vi "Güç_Tablo_Doldur.vi"(10 "Table Reference in":refnum<vi>, 11 "Array In":dbl[][](array[numeric])) -> (1 "Test Result":bool, 2 "Table Values":string[][](array[string]), 3 "Array Out":dbl[][](array[numeric]))   [LabVIEW 2014]
uses:
  TestStandInteraction/VeriPaylasim_Globali.vi
panel:
  out "OlcumNo":u16
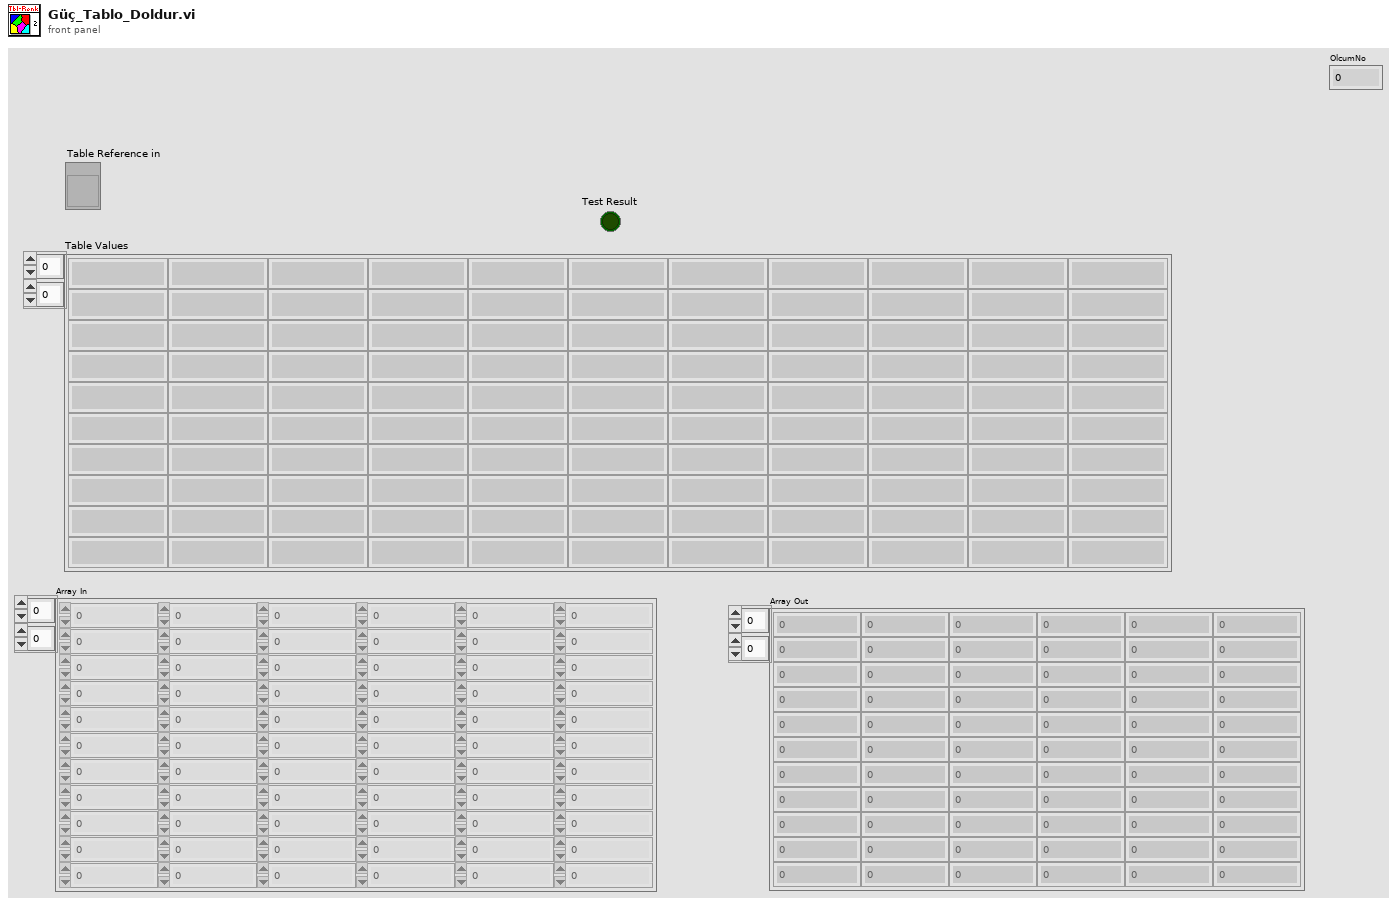
[diagram p1: front panel]
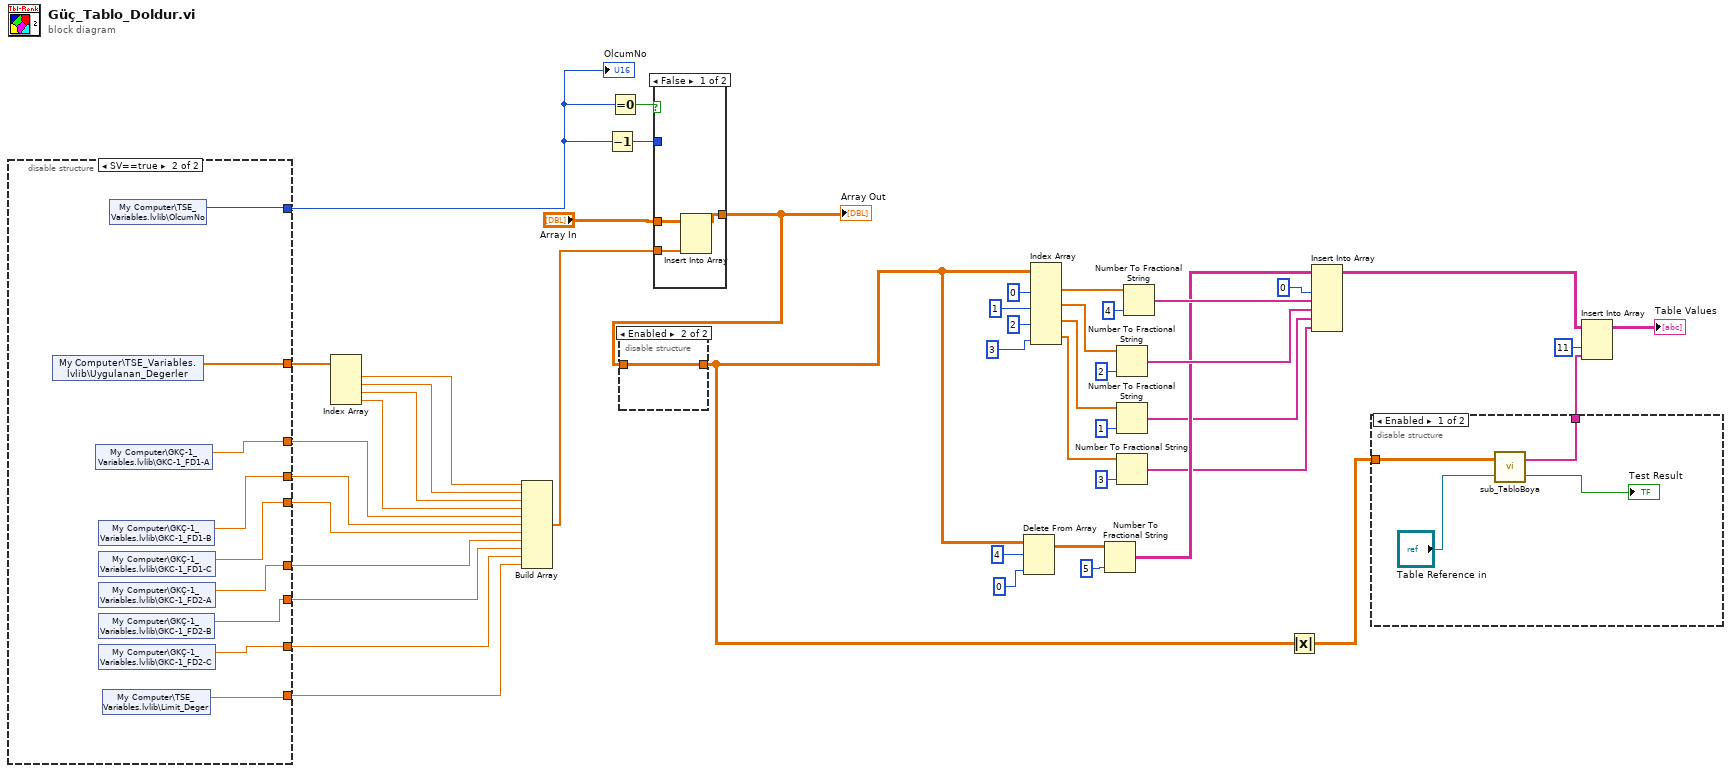
[diagram p0: block diagram]
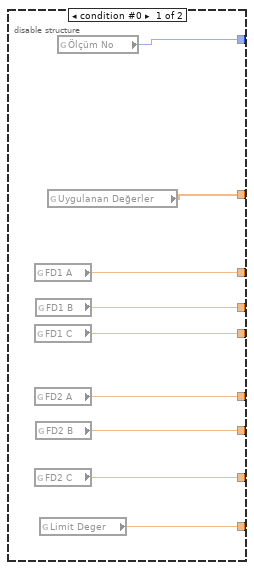
[diagram p2: hidden frame]
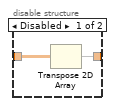
[diagram p3: hidden frame]
diagram:
  n1 = disable-structure shown="SV==true" {
    disable-tunnel: [w55 w57] -> w43
    disable-tunnel: [w54 w58] -> w8
    disable-tunnel: [w53 w59] -> w7
    disable-tunnel: [w52 w60] -> w6
    disable-tunnel: [w51 w61] -> w5
    disable-tunnel: [w50 w62] -> w4
    disable-tunnel: [w49 w63] -> w3
    disable-tunnel: [w48 w64] -> w2
    disable-tunnel: [w47 w56] -> w1
    frame condition #0 {
      n2 = global read "VeriPaylasim_Globali.vi" "FD1 A"() -> (w54:dbl)
      n3 = global read "VeriPaylasim_Globali.vi" "FD1 C"() -> (w52:dbl)
      n4 = global read "VeriPaylasim_Globali.vi" "FD2 A"() -> (w51:dbl)
      n5 = global read "VeriPaylasim_Globali.vi" "FD2 C"() -> (w49:dbl)
      n6 = global read "VeriPaylasim_Globali.vi" "FD1 B"() -> (w53:dbl)
      n7 = global read "VeriPaylasim_Globali.vi" "FD2 B"() -> (w50:dbl)
      n8 = global read "VeriPaylasim_Globali.vi" "Limit Deger"() -> (w48:dbl)
      n9 = global read "VeriPaylasim_Globali.vi" "Uygulanan Değerler"() -> (w55:dbl[])
      n10 = global read "VeriPaylasim_Globali.vi" "Ölçüm No"() -> (w47:u16)
    }
    frame condition #1 (active) {
      n11 = shared-variable "My Computer\\TSE_Variables.lvlib\\Uygulanan_Degerler"() -> (w57:dbl[])  [unwired: 1 in, 1 out]
      n12 = shared-variable "My Computer\\GKÇ-1_Variables.lvlib\\GKC-1_FD1-A"() -> (w58:dbl)  [unwired: 1 in, 1 out]
      n13 = shared-variable "My Computer\\GKÇ-1_Variables.lvlib\\GKC-1_FD1-B"() -> (w59:dbl)  [unwired: 1 in, 1 out]
      n14 = shared-variable "My Computer\\GKÇ-1_Variables.lvlib\\GKC-1_FD1-C"() -> (w60:dbl)  [unwired: 1 in, 1 out]
      n15 = shared-variable "My Computer\\GKÇ-1_Variables.lvlib\\GKC-1_FD2-A"() -> (w61:dbl)  [unwired: 1 in, 1 out]
      n16 = shared-variable "My Computer\\GKÇ-1_Variables.lvlib\\GKC-1_FD2-B"() -> (w62:dbl)  [unwired: 1 in, 1 out]
      n17 = shared-variable "My Computer\\GKÇ-1_Variables.lvlib\\GKC-1_FD2-C"() -> (w63:dbl)  [unwired: 1 in, 1 out]
      n18 = shared-variable "My Computer\\TSE_Variables.lvlib\\Limit_Deger"() -> (w64:dbl)  [unwired: 1 in, 1 out]
      n19 = shared-variable "My Computer\\TSE_Variables.lvlib\\OlcumNo"() -> (w56:u16)  [unwired: 1 in, 1 out]
    }
  }
  "OlcumNo" <- w1
  n20 = Index Array(array=w43) -> (element #1=w44:dbl, element #2=w37:dbl, element #3=w36:dbl, element #4=w35:dbl)  [unwired: 4 in]
  n21 = Build Array(w44, w37, w36, w35, w8, w7, w6, w5, w4, w3, w2) -> (w39:dbl[])
  n22 = Decrement(x=w1) -> (x-1=w41:u16)
  n23 = Equal To 0?(x=w1) -> (x = 0?=w42:bool)
  n24 = case shown="False" w42 {
    tunnel: w39 -> [w66 _]
    tunnel: [w65 w68] -> w38
    tunnel: "Array In" -> [w67 w68]
    tunnel: w41 -> [_ _]
    frame False {
      n25 = Insert Into Array(array=w67, new element=w66) -> (w65:dbl[][])  [unwired: 2 in]
    }
    frame True {
    }
  }
  "Array Out" <- w38
  n26 = disable-structure shown="Enabled" {
    disable-tunnel: w38 -> [w70 w71]
    disable-tunnel: [w69 w71] -> w27
    frame Disabled {
      n27 = Transpose 2D Array(2D array=w70) -> (transposed array=w69:dbl[][])
    }
    frame Enabled {
    }
  }
  n28 = Delete From Array "Delete From Array"(array=w27, length=4, index (col)=0 ("disabled index (col)")) -> (array with subset deleted=w24:dbl[][])  [unwired: 1 in, 1 out]
  n29 = Index Array "Index Array"(array=w27, index (col) #1=0 ("disabled index (col)"), index (col) #2=1 ("index (col)"), index (col) #3=2 ("index (col)"), index (col) #4=3 ("index (col)")) -> (element #1=w21:dbl[], element #2=w22:dbl[], element #3=w16:dbl[], element #4=w12:dbl[])  [unwired: 4 in]
  n30 = Number To Fractional String(number=w24, precision (6)=i16 5) -> (F-format string=w23:string[][])  [unwired: 2 in]
  n31 = Number To Fractional String(number=w22, precision (6)=i16 2) -> (F-format string=w28:string[])  [unwired: 2 in]
  n32 = Number To Fractional String(number=w16, precision (6)=i16 1) -> (F-format string=w15:string[])  [unwired: 2 in]
  n33 = Number To Fractional String(number=w12, precision (6)=i16 3) -> (F-format string=w11:string[])  [unwired: 2 in]
  n34 = Number To Fractional String(number=w21, precision (6)=i16 4) -> (F-format string=w32:string[])  [unwired: 2 in]
  n35 = Absolute Value(x=w27) -> (abs(x)=w9:dbl[][])
  n36 = Insert Into Array(array=w23, index (col)=0 ("disabled index (col)"), new element #1=w32, new element #2=w28, new element #3=w15, new element #4=w11) -> (w30:string[][])  [unwired: 1 in]
  n37 = disable-structure shown="Enabled" {
    disable-tunnel: w9 -> [w74 _]
    disable-tunnel: [w73 _] -> w46
    frame Enabled {
      n38 = call "sub_TabloBoya.vi"("Table in"="Table Reference in", "Tablo Degerleri"=w74) -> ("Test Result"=→"Test Result":bool, "RESULTS"=w73:string[])
    }
    frame Disabled {
    }
  }
  n39 = Insert Into Array(array=w30, index (col)=11 ("disabled index (col)"), new element=w46) -> (→"Table Values":string[][])  [unwired: 1 in]
